vi "add columns.vi"(10 "Old Col":string[](array[string]), 11 "New Col":string[](array[string])) -> (2 "为空？":bool, 3 "add col":string[](array[string]))   [LabVIEW 2016, in "SQLite Lib.lvlib"]
uses:
  SQLite Lib.lvlib
  <vilib>/regexp/Match Regular Expression.xnode
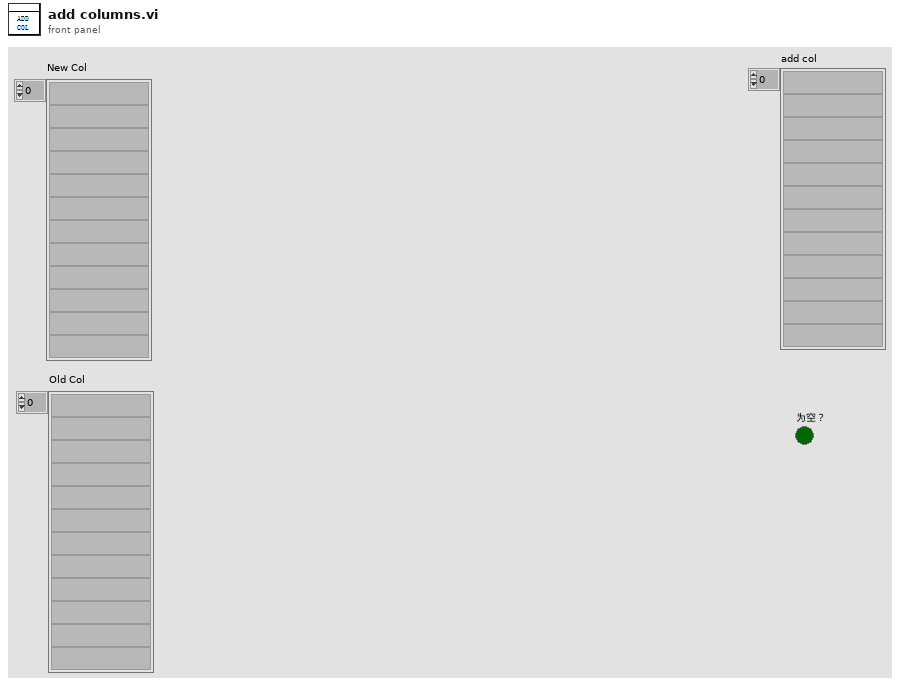
[diagram p1: front panel]
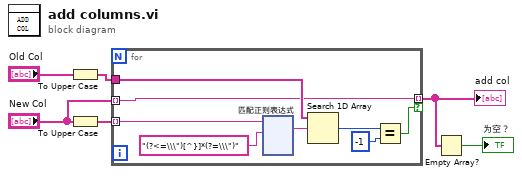
[diagram p0: block diagram]
diagram:
  n1 = To Upper Case(1:"Old Col") -> (0:w5:string[])
  n2 = To Upper Case(1:"New Col") -> (0:w4:string[])
  n3 = for {
    tunnel: w5 -> [w14]
    tunnel: w4 -> [w9] mode=indexing
    tunnel: [w10] -> w2 mode=indexing if=w11
    tunnel: "New Col" -> [w10] mode=indexing
    n4 = xnode "匹配正则表达式"("输入字符串"=w9, "正则表达式"="(?<=\\\")[^}]*(?=\\\")") -> ("所有匹配"=w7:string)  [unwired: 4 in, 4 out]
    n5 = Search 1D Array(1D array=w14, element=w7) -> (index of element=w13:i32)  [unwired: 1 in]
    n6 = Equal?(x=w13, y=-1) -> (x = y?=w11:bool)
  }
  "add col" <- w2
  n7 = Empty Array?(array=w2) -> (empty?=→"为空？":bool)
